vi "Decode Shooter Joystick.vi"(8 "reinitialize? (F)":bool) -> (0 "reinitialize":bool, 1 "full power":bool, 2 "Bottom RPM":dbl, 3 "Top RPM":dbl, 5 "firing":bool)   [LabVIEW 2011]
panel:
  in  "FULL POWER":bool
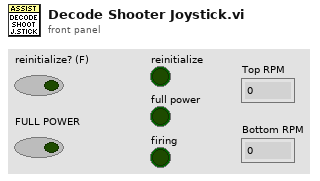
[diagram p1: front panel]
types:
  T1 = typedef "WPI_JoystickDevRef.ctl" = cluster{"Device":T2}
  T2 = typedef "WPI_JoystickDeviceEnum.ctl" = enum16{"USB 1", "USB 2", "USB 3", "USB 4", "Kinect 1", "Kinect 2"}
  T3 = typedef "WPI_JoystickButtonState.ctl" = cluster{"Button 1":bool, "Button 2":bool, "Button 3":bool, "Button 4":bool, "Button 5":bool, "Button 6":bool, "Button 7":bool, "Button 8":bool, "Button 9":bool, "Button 10":bool, "Button 11":bool, "Button 12":bool}
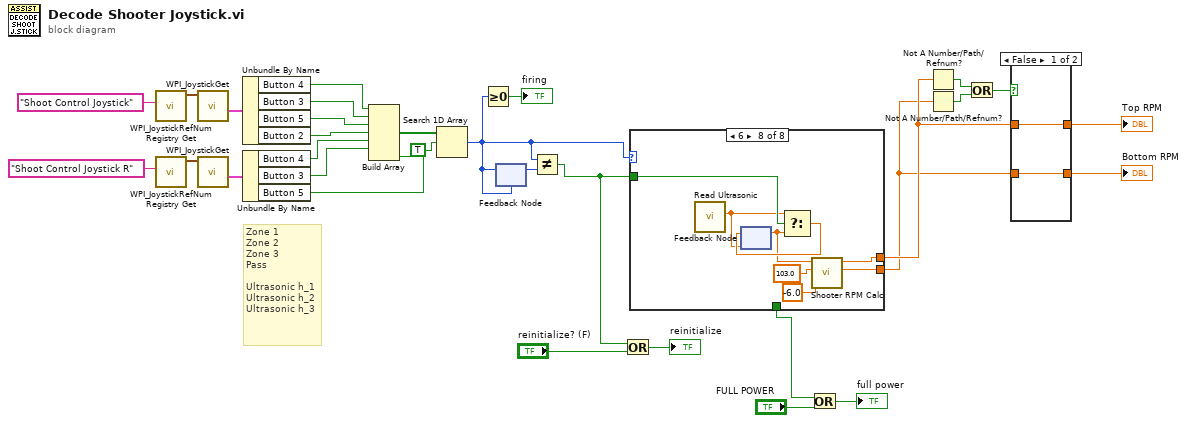
[diagram p0: block diagram]
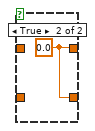
[diagram p2: hidden frame]
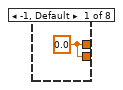
[diagram p3: hidden frame]
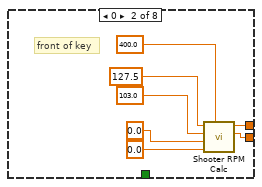
[diagram p4: hidden frame]
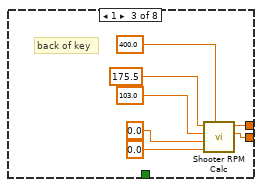
[diagram p5: hidden frame]
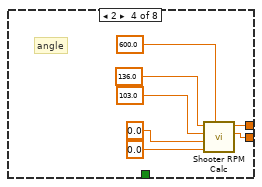
[diagram p6: hidden frame]
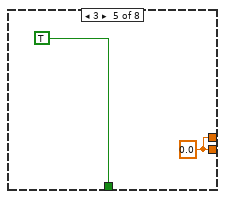
[diagram p7: hidden frame]
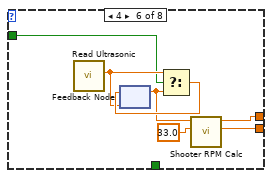
[diagram p8: hidden frame]
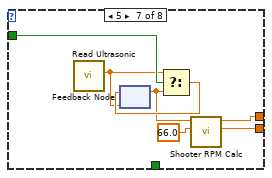
[diagram p9: hidden frame]
diagram:
  # "Zone 1\nZone 2\nZone 3\nPass\n\nUltrasonic h_1\nUltrasonic h_2\nUltrasonic h_3"
  n1 = call <vilib>:"WPI_JoystickRefNum Registry Get.vi"("refnum name"="Shoot Control Joystick") -> ("JoystickDevRef"=w30:T1)  [unwired: 9 in, 1 out]
  n2 = call <vilib>:"WPI_JoystickRefNum Registry Get.vi"("refnum name"="Shoot Control Joystick R") -> ("JoystickDevRef"=w27:T1)  [unwired: 9 in, 1 out]
  n3 = call <vilib>:"WPI_JoystickGet.vi"("JoystickDevRef"=w30) -> ("Buttons"=w29:T3)  [unwired: 4 in, 2 out]
  n4 = call <vilib>:"WPI_JoystickGet.vi"("JoystickDevRef"=w27) -> ("Buttons"=w25:T3)  [unwired: 4 in, 2 out]
  n5 = Unbundle By Name(w29) -> ("Button 4"=w24:bool, "Button 3"=w23:bool, "Button 5"=w22:bool, "Button 2"=w21:bool)
  n6 = Unbundle By Name(w25) -> ("Button 4"=w19:bool, "Button 3"=w18:bool, "Button 5"=w17:bool)
  n7 = Build Array(w24, w23, w22, w21, w19, w18, w17) -> (w28:bool[])
  n8 = Search 1D Array(1D array=w28, element=TRUE) -> (index of element=w6:i32)  [unwired: 1 in]
  n9 = Greater Or Equal To 0?(x=w6) -> (x >= 0?=→"firing":bool)
  n10 = feedback #1(w6) -> (w14:i32)
  n11 = feedback-in #1(w6) -> ()
  n12 = Not Equal?(x=w6, y=w14) -> (x != y?=w5:bool)
  n13 = Or(x=w5, y="reinitialize? (F)") -> (x .or. y?=→"reinitialize":bool)
  n14 = case shown="6" w6 {
    tunnel: [w32 w39 w46 w53 w55 w56 w64 w71] -> w15
    tunnel: [w32 w38 w45 w52 w55 w60 w63 w72] -> w8
    tunnel: w5 -> [_ _ _ _ _ w57 w68 w76]
    tunnel: [_ _ _ _ TRUE _ _ _] -> w7
    frame -1, Default {
      w32 = 0.0 ("Top RPM")
    }
    frame 0 {
      # "front of key"
      n15 = call "Shooter RPM Calc.vi"("Backspin"=400.0 ("backspin"), "Height Trim"=0.0 ("h trim"), "Distance Trim"=0.0 ("d trim"), "Height"=103.0 ("Distance"), "Distance"=127.5 ("Height")) -> ("Bottom RPM"=w38:dbl, "Top RPM"=w39:dbl)  [unwired: 4 in, 1 out]
    }
    frame 1 {
      # "back of key"
      n16 = call "Shooter RPM Calc.vi"("Backspin"=400.0 ("backspin"), "Height Trim"=0.0 ("h trim"), "Distance Trim"=0.0 ("d trim"), "Height"=103.0 ("Distance"), "Distance"=175.5 ("Height")) -> ("Bottom RPM"=w45:dbl, "Top RPM"=w46:dbl)  [unwired: 4 in, 1 out]
    }
    frame 2 {
      # "angle"
      n17 = call "Shooter RPM Calc.vi"("Backspin"=600.0 ("backspin"), "Height Trim"=0.0 ("h trim"), "Distance Trim"=0.0 ("d trim"), "Height"=103.0 ("Distance"), "Distance"=136.0 ("Height")) -> ("Bottom RPM"=w52:dbl, "Top RPM"=w53:dbl)  [unwired: 4 in, 1 out]
    }
    frame 3 {
      w55 = 0.0 ("Bottom RPM")
    }
    frame 4 {
      n18 = call "Read Ultrasonic.vi"() -> ("distance"=w61:dbl)  [unwired: 11 in]
      n19 = feedback #2(w61) -> (w59:dbl)
      n20 = Select(t=w61, s=w57, f=w59) -> (s? t:f=w62:dbl)
      n21 = feedback-in #2(w62) -> ()
      n22 = call "Shooter RPM Calc.vi"("Height"=33.0, "Distance"=w59) -> ("Bottom RPM"=w60:dbl, "Top RPM"=w56:dbl)  [unwired: 7 in, 1 out]
    }
    frame 5 {
      n23 = call "Read Ultrasonic.vi"() -> ("distance"=w67:dbl)  [unwired: 11 in]
      n24 = feedback #3(w67) -> (w66:dbl)
      n25 = Select(t=w67, s=w68, f=w66) -> (s? t:f=w69:dbl)
      n26 = feedback-in #3(w69) -> ()
      n27 = call "Shooter RPM Calc.vi"("Height"=66.0, "Distance"=w66) -> ("Bottom RPM"=w63:dbl, "Top RPM"=w64:dbl)  [unwired: 7 in, 1 out]
    }
    frame 6 {
      n28 = call "Read Ultrasonic.vi"() -> ("distance"=w75:dbl)  [unwired: 11 in]
      n29 = feedback #4(w75) -> (w74:dbl)
      n30 = Select(t=w75, s=w76, f=w74) -> (s? t:f=w77:dbl)
      n31 = feedback-in #4(w77) -> ()
      n32 = call "Shooter RPM Calc.vi"("Height Trim"=-6.0, "Height"=103.0, "Distance"=w74) -> ("Bottom RPM"=w72:dbl, "Top RPM"=w71:dbl)  [unwired: 6 in, 1 out]
    }
  }
  n33 = Or(x=w7, y="FULL POWER") -> (x .or. y?=→"full power":bool)
  n34 = Not A Number/Path/Refnum?(number/path/refnum=w15) -> (NaN/Path/Refnum?=w11:bool)
  n35 = Not A Number/Path/Refnum?(number/path/refnum=w8) -> (NaN/Path/Refnum?=w16:bool)
  n36 = Or(x=w11, y=w16) -> (x .or. y?=w10:bool)
  n37 = case shown="False" w10 {
    tunnel: [w78 w80] -> w1
    tunnel: [w79 w80] -> w2
    tunnel: w15 -> [w79 _]
    tunnel: w8 -> [w78 _]
    frame False {
    }
    frame True {
      w80 = 0.0
    }
  }
  "Top RPM" <- w2
  "Bottom RPM" <- w1
